vi "TEST_INTERPOLATE_ROTATION.vi"() -> ()   [LabVIEW 2023]
uses:
  <vilib>/Rock Robotics/WPI/ThirdParty/JAS_Junk/TrajLib/TypeDef/ROTATION2D.ctl
  <vilib>/Rock Robotics/WPI/ThirdParty/JAS_Junk/TrajLib/Trajectory_Library.lvlib
panel:
  out "Elaspsed Traj Time Sec":dbl
  out "Orientation Demand":T1 {"SIN" format="%13.4f"; "COS" format="%13.4f"; "VALUE" format="%13.4f"}
  out "Orientation Demand Deg":dbl
  out "Rotational Velocity Rad Per Sec":dbl
  in  "Starting Orientation  DEG":dbl=-179.0
  in  "End Orientation Demand DEG":dbl=120.0
  in  "Total Trajectory Time Sec":dbl=10.0
  in  "Completion Fraction":dbl=0.75
  in  "Init":bool
  in  "Starting Fraction":dbl=0.25
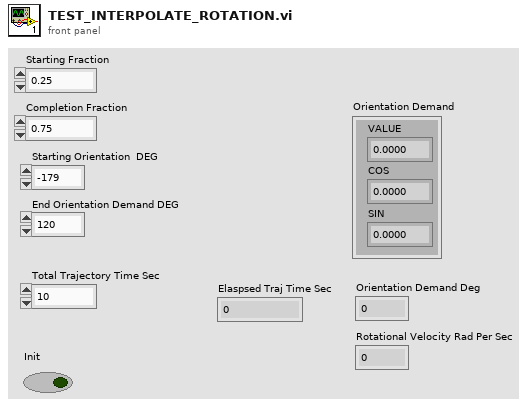
[diagram p1: front panel]
types:
  T1 = typedef "Trajectory_Library.lvlib/ROTATION2D.ctl" = cluster{"VALUE":dbl, "COS":dbl, "SIN":dbl}
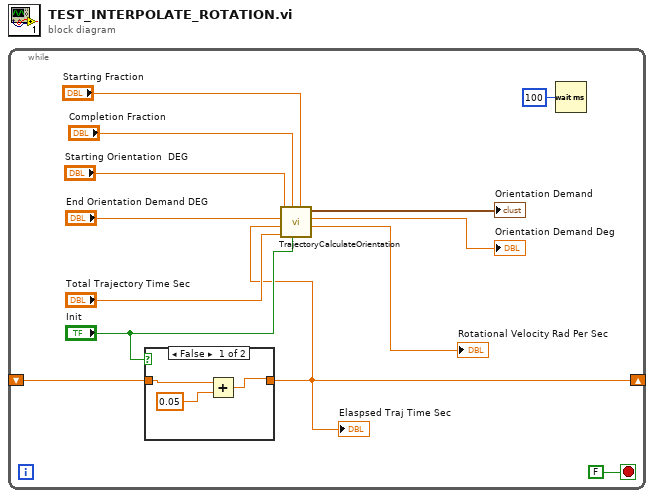
[diagram p0: block diagram]
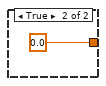
[diagram p2: hidden frame]
diagram:
  n1 = while {
    shift-right: [w1] -> _
    shift-left: _ -> [w3]
    stop <- FALSE stop-if-true
    n2 = case shown="False" "Init" {
      tunnel: [w15 0.0] -> w1
      tunnel: w3 -> [w16 _]
      frame False {
        n3 = Add(x=w16, y=0.05) -> (x+y=w15:dbl)
      }
      frame True {
      }
    }
    "Elaspsed Traj Time Sec" <- w1
    n4 = call "TrajectoryCalculateOrientation.vi"("Starting Fraction"="Starting Fraction", "Init"="Init", "Completion Fraction"="Completion Fraction", "Total Trajectory Time Sec"="Total Trajectory Time Sec", "Elapsed Traj Time Sec"=w1, "End Orientation Demand DEG"="End Orientation Demand DEG", "Starting Orientation  DEG"="Starting Orientation  DEG") -> ("Rotational Velocity Rad Per Sec"=→"Rotational Velocity Rad Per Sec":dbl, "Orientation Demand Deg"=→"Orientation Demand Deg":dbl, "Orientation Demand"=→"Orientation Demand":T1)  [unwired: 2 in]
    n5 = Wait (ms)(milliseconds to wait=u32 100) -> ()  [unwired: 1 out]
  }
